vi "Initialize DO.vi"(8 "error in (no error)":errorcluster, 9 "DO Channel Setting":T1, 10 "DAQ Type":enum16{"Hardware", "Simulation"}(ring), 11 "PXIe 6363 in":refnum<class "PXIe 6363.lvclass">) -> (0 "error out":errorcluster, 3 "PXIe 6363 out":refnum<class "PXIe 6363.lvclass">)   [LabVIEW 2016, in "DAQ Hardware.lvlib" / "PXIe 6363.lvclass"]
uses:
  PXIe 6363.lvclass
  DO Channel Setting.ctl
  PXIe 6363.lvclass/PXIe 6363.ctl
  DAQ Hardware.lvlib
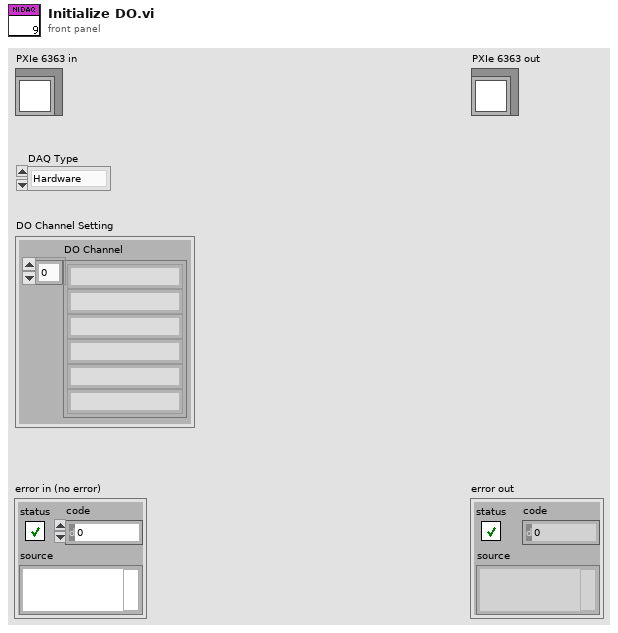
[diagram p1: front panel]
types:
  T1 = typedef "DAQ Hardware.lvlib/DO Channel Setting.ctl" = cluster{"DO Channel":string[]}
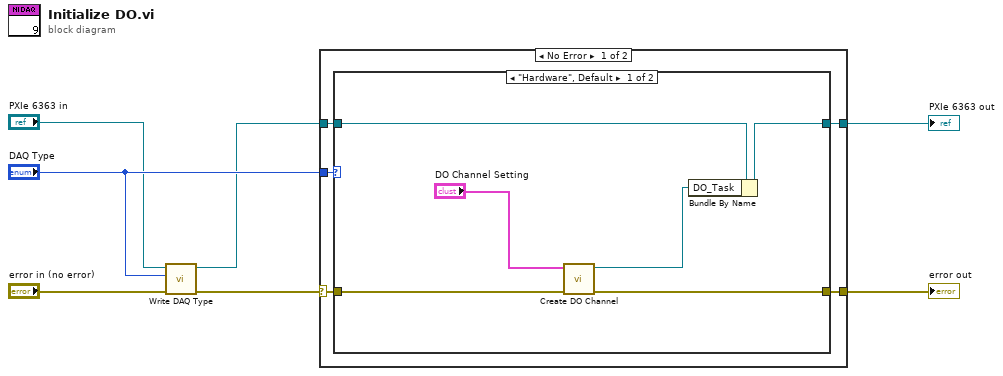
[diagram p0: block diagram]
diagram:
  n1 = call-dynamic "Write DAQ Type.vi"("error in (no error)"="error in (no error)", "DAQ Type"="DAQ Type", "PXIe 6363 in"="PXIe 6363 in") -> ("error out"=w6:errorcluster, "PXIe 6363 out"=w1:refnum<class "PXIe 6363.lvclass">)  [unwired: 7 in]
  n2 = case shown="No Error" w6 {
    selector: w6 -> [w11 w21]
    tunnel: "DAQ Type" -> [w12 _]
    tunnel: w1 -> [w10 w22]
    tunnel: [w9 w22] -> w3
    tunnel: [w8 w21] -> w2
    frame No Error {
      n3 = case shown="\"Hardware\", Default" w12 {
        tunnel: w11 -> [w18 w19]
        tunnel: w10 -> [w17 w20]
        tunnel: [w15 w20] -> w9
        tunnel: [w16 w19] -> w8
        frame "Hardware", Default {
          n4 = call "Create DO Channel.vi"("error in (no error)"=w18, "DO Channel Setting"="DO Channel Setting") -> ("error out"=w16:errorcluster, "DO_Task"=w13:refnum<k21>)  [unwired: 8 in]
          n5 = Bundle By Name(cluster=w17, "DO_Task"=w13) -> (w15:refnum<class "PXIe 6363.lvclass">)
        }
        frame "Simulation" {
        }
      }
    }
    frame Error {
    }
  }
  "error out" <- w2
  "PXIe 6363 out" <- w3
